vi "Bundle_saving_buffer.vi"(5 "File saving directory/folder":path, 6 "new element/subarray":dbl[](array[numeric]), 7 "Conc cases start @ 0":dbl, 8 "Boolean":bool, 9 "Numeric":dbl, 10 "Array":dbl[][](array[numeric]), 11 "Intitializer Value":dbl) -> (2 "Intitializer Value 2":dbl)   [LabVIEW 2021]
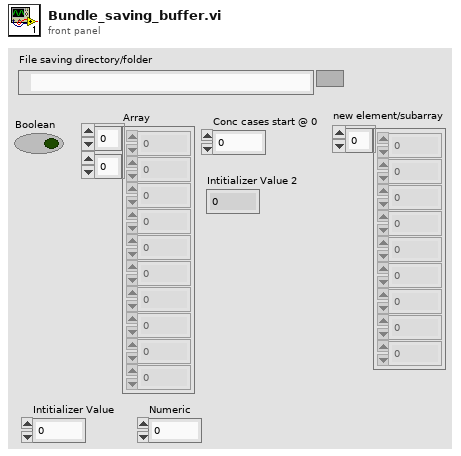
[diagram p1: front panel]
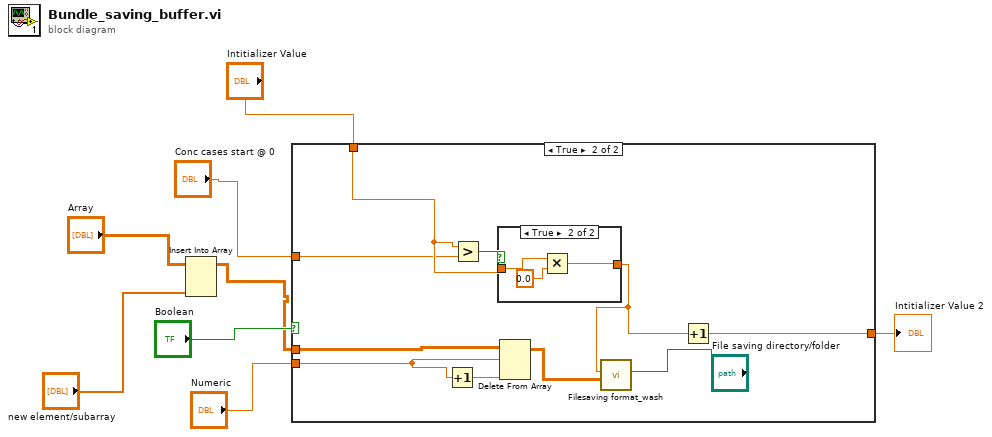
[diagram p0: block diagram]
diagram:
  n1 = Insert Into Array(array="Array", new element="new element/subarray") -> (w1:dbl[][])  [unwired: 2 in]
  n2 = case shown="True" "Boolean" {
    tunnel: [w9 w19] -> w6
    tunnel: "Intitializer Value" -> [w9 w15]
    tunnel: w1 -> [_ w18]
    tunnel: "Numeric" -> [_ w17]
    tunnel: "Conc cases start @ 0" -> [_ w13]
    frame False {
    }
    frame True {
      n3 = Increment(x=w17) -> (x+1=w16:dbl)
      n4 = Greater?(x=w15, y=w13) -> (0:w14:bool)
      n5 = case shown="True" w14 {
        tunnel: w15 -> [w20 w23]
        tunnel: [w20 w21] -> w12
        frame False {
        }
        frame True {
          n6 = Multiply(x=w23, y=0.0) -> (x*y=w21:dbl)
        }
      }
      n7 = Delete From Array(array=w18, length=w17, index (col)=w16) -> (array with subset deleted=w11:dbl[][])  [unwired: 1 in, 1 out]
      n8 = call "Filesaving format_wash.vi"("base path"="File saving directory/folder", "2D data"=w11, "Numeric"=w12) -> ()  [unwired: 9 in]
      n9 = Increment(x=w12) -> (x+1=w19:dbl)
    }
  }
  "Intitializer Value 2" <- w6
